vi "SetTemplate.vi"(8 "error in (no error)":errorcluster, 10 "Set_Val":i32, 11 "OneOfTemplate in":refnum<class "OneOfTemplate.lvclass">) -> (0 "error out":errorcluster, 3 "OneOfTemplate out":refnum<class "OneOfTemplate.lvclass">)   [LabVIEW 2019, in "OneOfTemplate.lvclass"]
uses:
  <vilib>/gRPC/gRPC Server and Client Template [2]/Oneof Template/OneOfTemplate.lvclass
  <vilib>/gRPC/gRPC Server and Client Template [2]/Oneof Template/OneOfTemplate.lvclass/OneOfTemplate.ctl
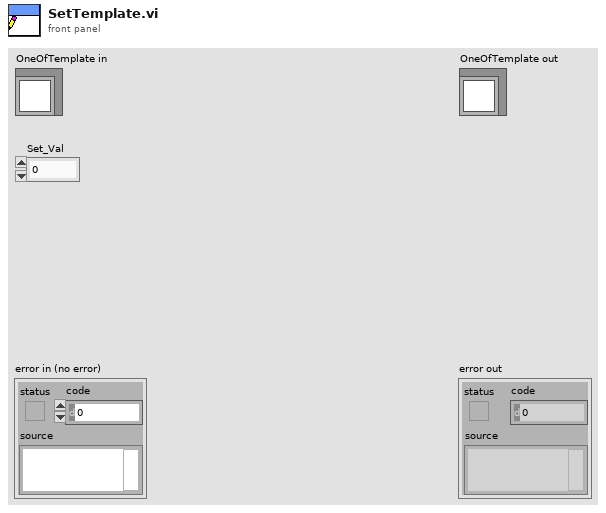
[diagram p1: front panel]
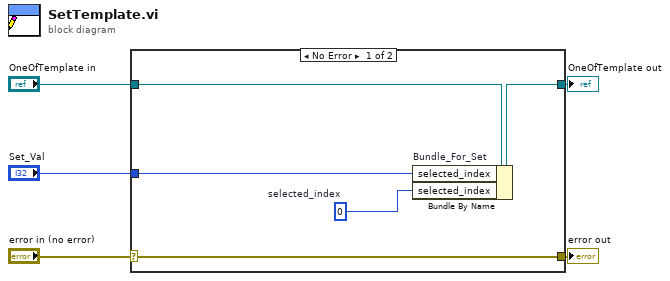
[diagram p0: block diagram]
diagram:
  n1 = case shown="No Error" "error in (no error)" {
    selector: "error in (no error)" -> [w10 w11]
    tunnel: [w10 w11] -> w4
    tunnel: [w8 w12] -> w2
    tunnel: "OneOfTemplate in" -> [w9 w12]
    tunnel: "Set_Val" -> [w7 _]
    frame No Error {
      w6 = 0  # selected_index
      n2 = Bundle By Name "Bundle_For_Set"(cluster=w9, "selected_index"=w7, "selected_index"=w6) -> (w8:refnum<class "OneOfTemplate.lvclass">)
    }
    frame Error {
    }
  }
  "error out" <- w4
  "OneOfTemplate out" <- w2
